vi "semicolon_delimited_string_to_points.vi"(11 "delimited string":string) -> (3 "Array":cluster{"X":dbl, "Y":dbl}[](array[cluster]))   [LabVIEW 2019]
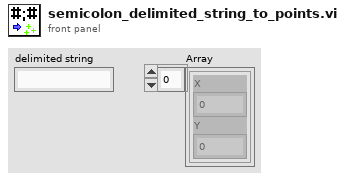
[diagram p1: front panel]
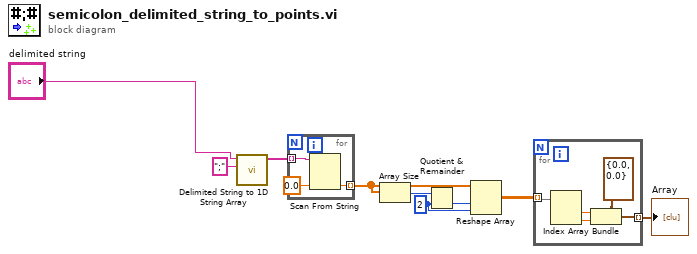
[diagram p0: block diagram]
diagram:
  w7 = 2 ("y")
  n1 = call <vilib>:"Delimited String to 1D String Array.vi"("delimiter"=";", "delimited string"="delimited string") -> ("string array"=w3:string[])  [unwired: 9 in]
  n2 = for {
    tunnel: w3 -> [w12] mode=indexing
    tunnel: [w10] -> w4 mode=indexing
    n3 = Scan From String(input string=w12, default 1=0.0 ("default value 1")) -> (output 1=w10:dbl)  [unwired: 3 in, 3 out]
  }
  n4 = Array Size(array=w4) -> (size(s)=w5:i32)
  n5 = Quotient & Remainder(x=w5, y=w7) -> (floor(x/y)=w6:i32)  [unwired: 1 out]
  n6 = Reshape Array(w4, w6, w7) -> (w8:dbl[][])
  n7 = for {
    tunnel: w8 -> [w16] mode=indexing
    tunnel: [w13] -> w9 mode=indexing
    n8 = Index Array(array=w16) -> (element #1=w15:dbl, element #2=w14:dbl)  [unwired: 2 in]
    n9 = Bundle(cluster=cluster{"X":dbl, "Y":dbl} {"X"=0.0, "Y"=0.0}, "X"=w15, "Y"=w14) -> (w13:cluster{"X":dbl, "Y":dbl})
  }
  "Array" <- w9
